vi "GetIQ_int16.vi"(8 "error in (no error)":errorcluster, 11 "reference in":refnum<class "IQBurst_memo.lvclass">) -> (0 "error out":errorcluster, 1 "dt":dbl, 2 "data":i16[](array[numeric]), 3 "reference out":refnum<class "IQBurst_memo.lvclass">)   [LabVIEW 2019, in "IQBurst_memo.lvclass"]
uses:
  IQBurst_memo.lvclass
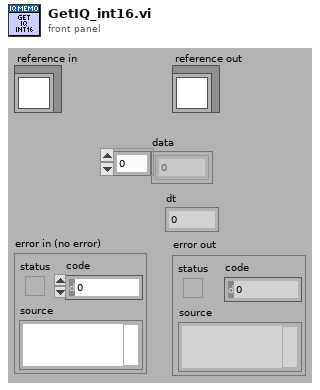
[diagram p1: front panel]
types:
  T1 = typedef "IQBurst_memo.lvclass/ObjectAttributes.ctl" = cluster{"IQ data":i16[], "dt":dbl}
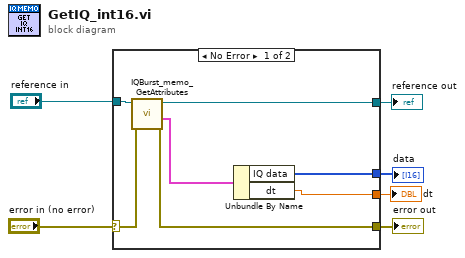
[diagram p0: block diagram]
diagram:
  n1 = case shown="No Error" "error in (no error)" {
    selector: "error in (no error)" -> [w13 w15]
    tunnel: [w12 w15] -> w5
    tunnel: [w11 w14] -> w3
    tunnel: "reference in" -> [w9 w14]
    tunnel: [w8 _] -> w2
    tunnel: [w7 _] -> w1
    frame No Error {
      n2 = call "IQBurst_memo_GetAttributes.vi"("error in (no error)"=w13, "reference in"=w9) -> ("error out"=w12:errorcluster, "attributes"=w10:T1, "reference out"=w11:refnum<class "IQBurst_memo.lvclass">)  [unwired: 6 in, 1 out]
      n3 = Unbundle By Name(w10) -> ("IQ data"=w8:i16[], "dt"=w7:dbl)
    }
    frame Error {
    }
  }
  "error out" <- w5
  "reference out" <- w3
  "data" <- w2
  "dt" <- w1
